vi "EDS test 01_with motor and Firebase with all sensors.vi"() -> ()   [LabVIEW 2020]
uses:
  <vilib>/DAQmx/read.llb/DAQmx Read (Digital Bool 1Line 1Point).vi
  <vilib>/DAQmx/write.llb/DAQmx Write (Digital Bool 1Line 1Point).vi
  <vilib>/DAQmx/read.llb/DAQmx Read (Analog Wfm 1Chan 1Samp).vi
  <vilib>/Analysis/baseanly.llb/Mean (DBL).vi
  <vilib>/Instr/_visa.llb/VISA Configure Serial Port (Instr).vi
  <vilib>/DAQmx/create/channels.llb/DAQmx Create Channel (DI-Digital Input).vi
  <vilib>/DAQmx/create/channels.llb/DAQmx Create Channel (DO-Digital Output).vi
  <vilib>/DAQmx/create/channels.llb/DAQmx Create Channel (AI-Voltage-Basic).vi
  <vilib>/DAQmx/miscellaneous.llb/DAQmx Fill In Error Info.vi
  <vilib>/httpClient/PUTBuffer.vi
  <vilib>/httpClient/LabVIEWHTTPClient.lvlib
  <vilib>/Analysis/NI_AALBase.lvlib
panel:
  out "Custom Sensor * 25":dbl(graph)
  out "Custom Sensor":dbl
  out "Train Speed":string
  out "Trolley Speed":string
  out "Trolley Distance":dbl
  out "Elephant Distance":dbl
  out "IR and Force Sensor":bool
  out "Custom Sensor":waveform(dbl)(graph)
  out "error out":errorcluster
  out "Concatenated String":string
  out "read buffer":string
  in  "stop":bool
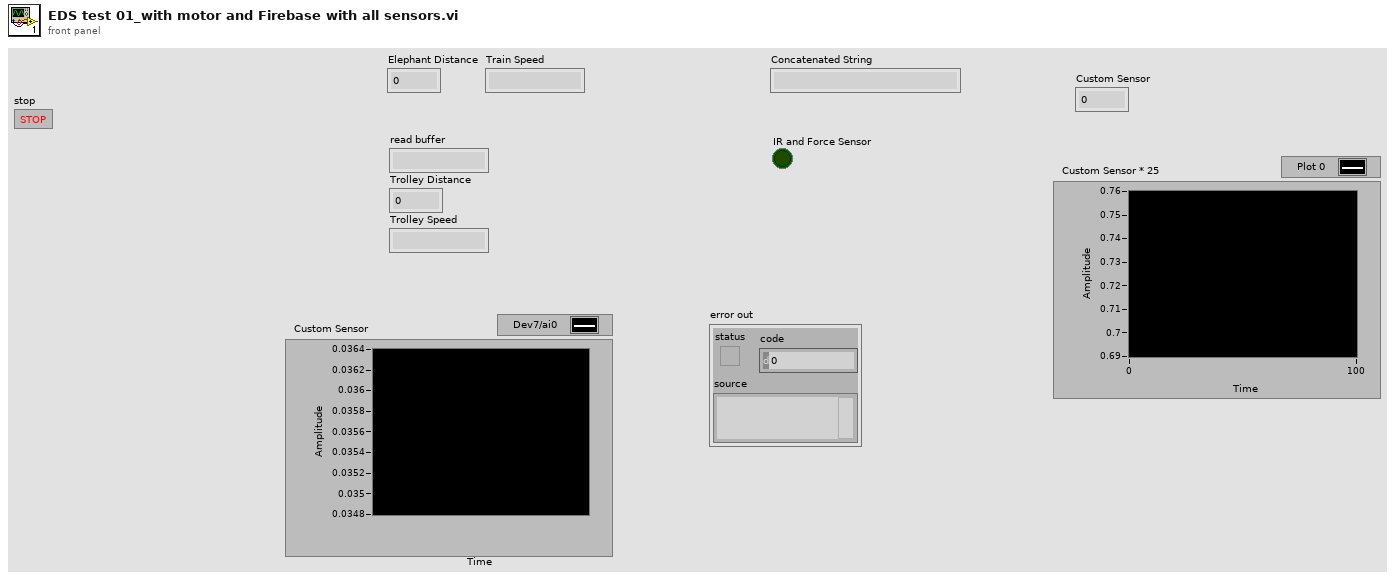
[diagram p1: front panel]
types:
  T1 = typedef "LabVIEWHTTPClient.lvlib/ClientHandle.ctl" = refnum<k1>
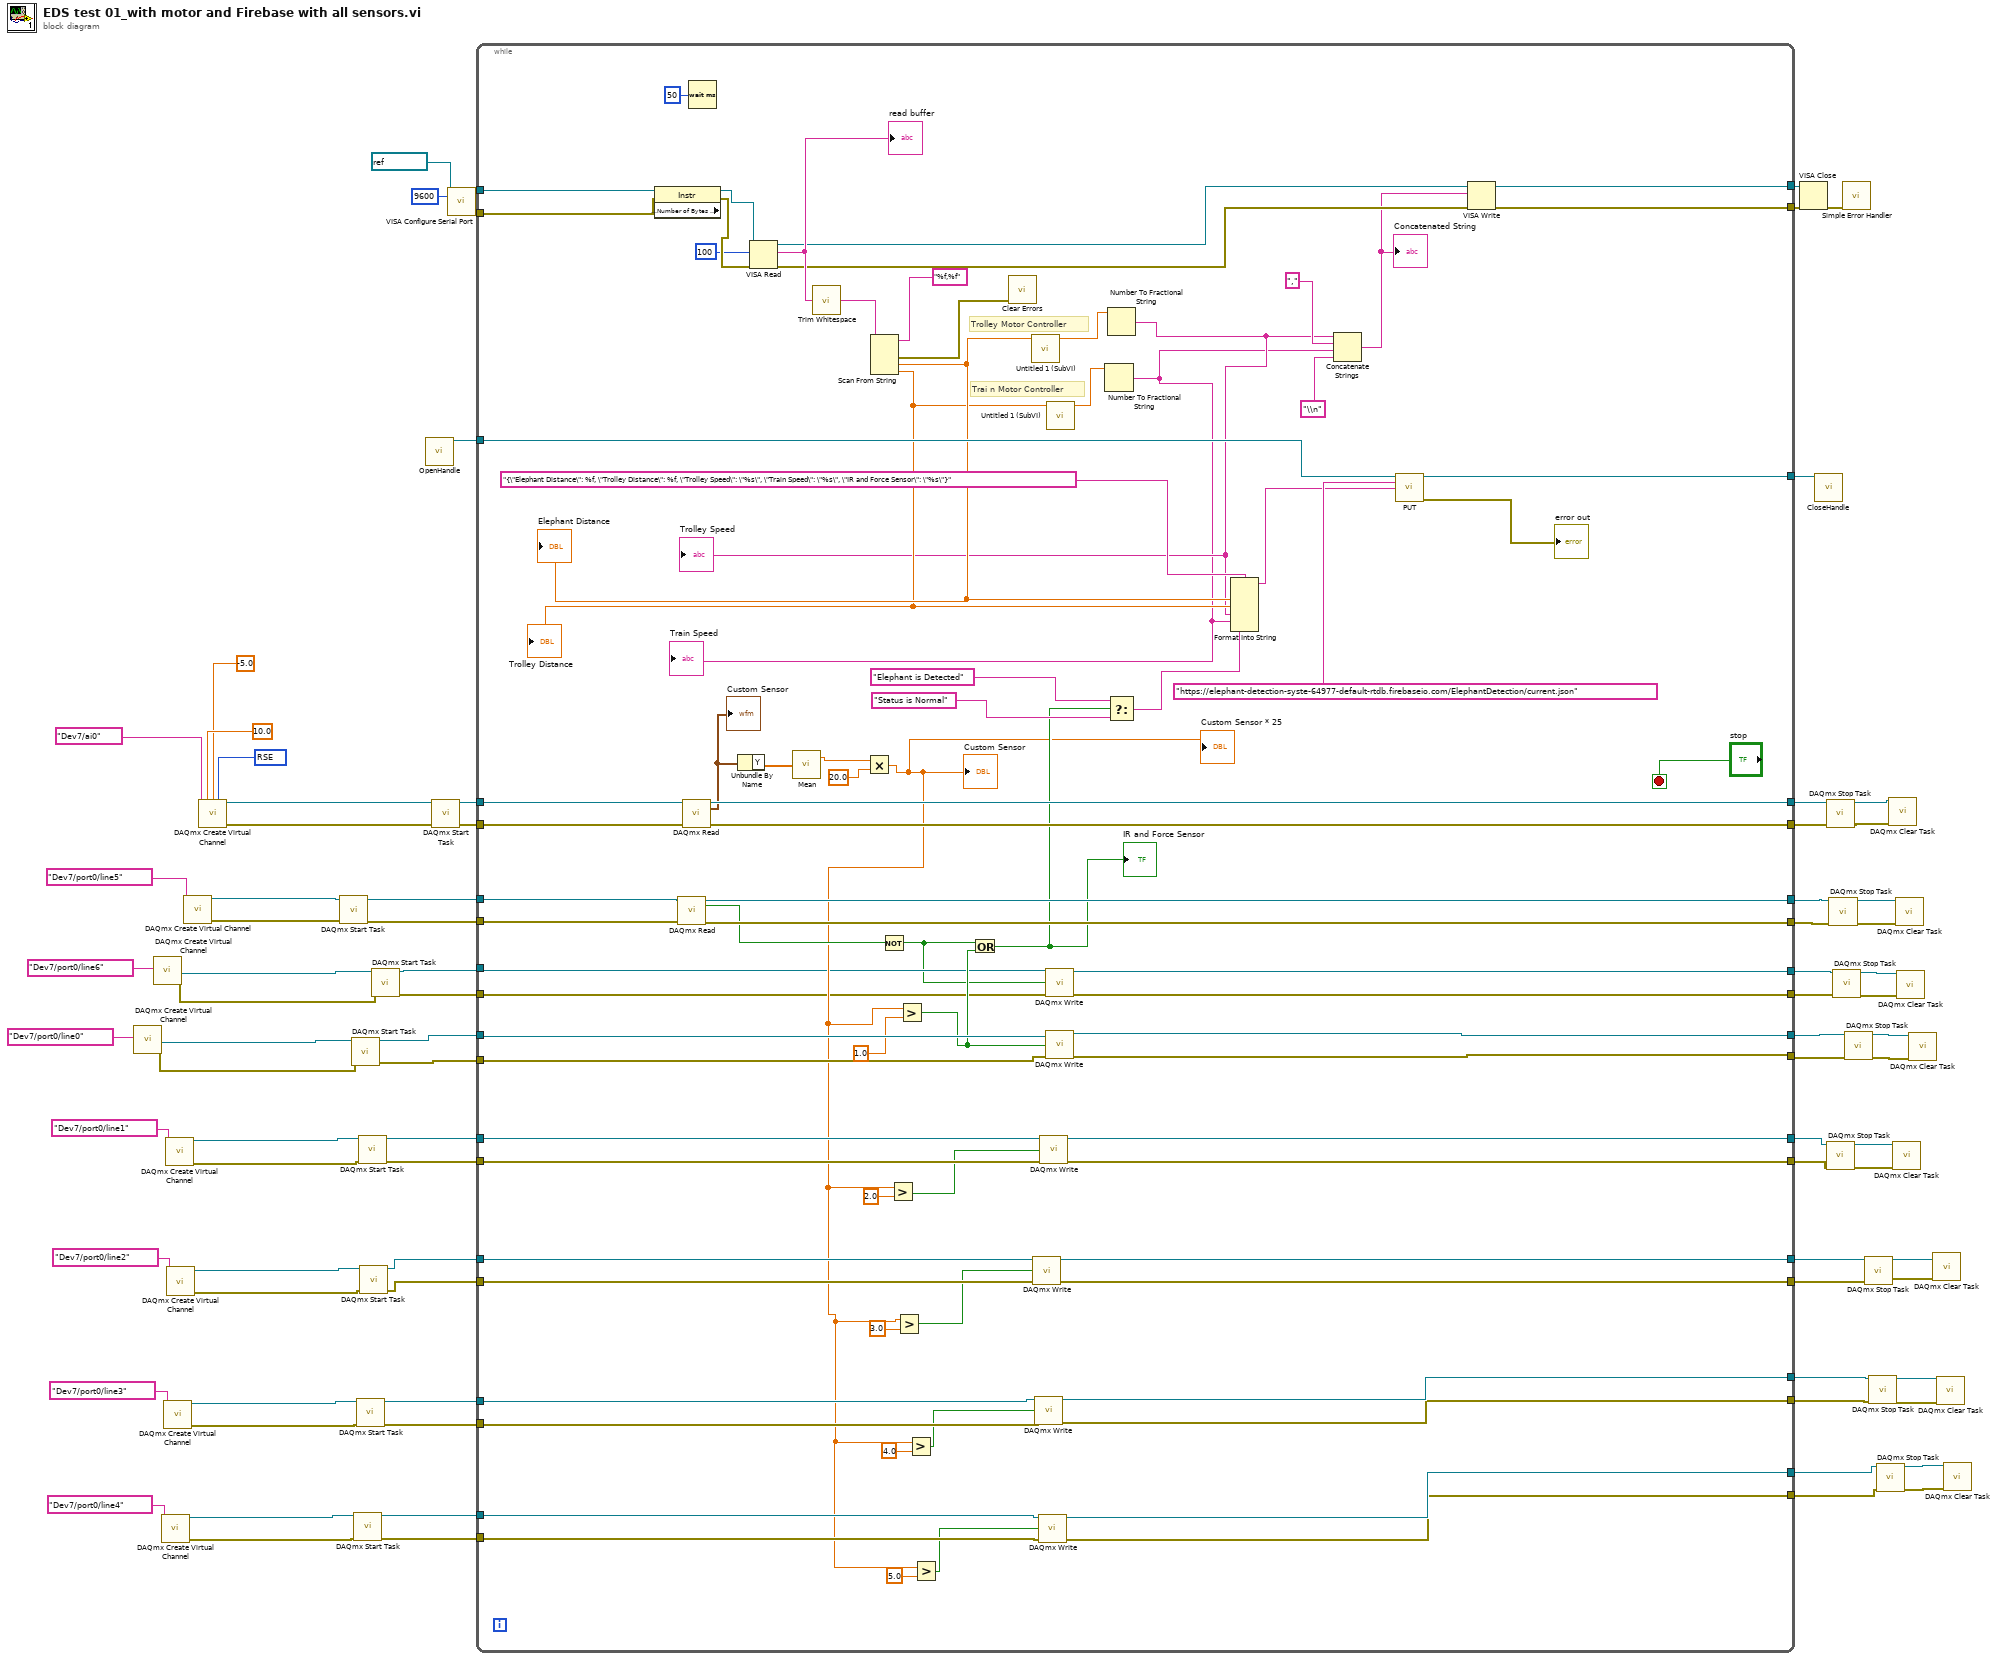
[diagram p0: block diagram]
diagram:
  w48 = 10083 items=["Default"=-1, "RSE"=10083, "NRSE"=10078, "Differential"=10106, "Pseudodifferential"=12529] ("input terminal configuration")
  n1 = call-poly <vilib>:"DAQmx Create Virtual Channel.vi"("lines"=tag "Dev7/port0/line0") -> ("task out"=w57:refnum<k21>, "error out"=w55:errorcluster)  [unwired: 13 in]
  n2 = call-poly <vilib>:"DAQmx Create Virtual Channel.vi"("lines"=tag "Dev7/port0/line6") -> ("task out"=w9:refnum<k21>, "error out"=w8:errorcluster)  [unwired: 13 in]
  n3 = call-poly <vilib>:"DAQmx Create Virtual Channel.vi"("lines"=tag "Dev7/port0/line4") -> ("task out"=w24:refnum<k21>, "error out"=w23:errorcluster)  [unwired: 13 in]
  n4 = call-poly <vilib>:"DAQmx Create Virtual Channel.vi"("lines"=tag "Dev7/port0/line3") -> ("task out"=w27:refnum<k21>, "error out"=w26:errorcluster)  [unwired: 13 in]
  n5 = call-poly <vilib>:"DAQmx Create Virtual Channel.vi"("lines"=tag "Dev7/port0/line1") -> ("task out"=w47:refnum<k21>, "error out"=w46:errorcluster)  [unwired: 13 in]
  n6 = call-poly <vilib>:"DAQmx Create Virtual Channel.vi"("lines"=tag "Dev7/port0/line2") -> ("task out"=w44:refnum<k21>, "error out"=w43:errorcluster)  [unwired: 13 in]
  n7 = call-poly <vilib>:"DAQmx Create Virtual Channel.vi"("lines"=tag "Dev7/port0/line5") -> ("task out"=w65:refnum<k21>, "error out"=w64:errorcluster)  [unwired: 13 in]
  n8 = call-poly <vilib>:"DAQmx Create Virtual Channel.vi"("maximum value"=10.0, "minimum value"=-5.0, "input terminal configuration"=w48, "physical channels"=tag "Dev7/ai0") -> ("task out"=w29:refnum<k21>, "error out"=w28:errorcluster)  [unwired: 10 in]
  n9 = call <vilib>:"DAQmx Start Task.vi"("task/channels in"=w65, "error in"=w64) -> ("task out"=w63:refnum<k21>, "error out"=w62:errorcluster)  [unwired: 12 in]
  n10 = call <vilib>:"DAQmx Start Task.vi"("task/channels in"=w57, "error in"=w55) -> ("task out"=w56:refnum<k21>, "error out"=w54:errorcluster)  [unwired: 12 in]
  n11 = call <vilib>:"DAQmx Start Task.vi"("task/channels in"=w24, "error in"=w23) -> ("task out"=w11:refnum<k21>, "error out"=w10:errorcluster)  [unwired: 12 in]
  n12 = call <vilib>:"DAQmx Start Task.vi"("task/channels in"=w27, "error in"=w26) -> ("task out"=w13:refnum<k21>, "error out"=w12:errorcluster)  [unwired: 12 in]
  n13 = call <vilib>:"DAQmx Start Task.vi"("task/channels in"=w47, "error in"=w46) -> ("task out"=w41:refnum<k21>, "error out"=w40:errorcluster)  [unwired: 12 in]
  n14 = call <vilib>:"DAQmx Start Task.vi"("task/channels in"=w44, "error in"=w43) -> ("task out"=w39:refnum<k21>, "error out"=w38:errorcluster)  [unwired: 12 in]
  n15 = call <vilib>:"DAQmx Start Task.vi"("task/channels in"=w9, "error in"=w8) -> ("task out"=w6:refnum<k21>, "error out"=w5:errorcluster)  [unwired: 12 in]
  n16 = call <vilib>:"OpenHandle.vi"() -> ("client handle out"=w77:T1)  [unwired: 14 in, 1 out]
  n17 = call <vilib>:"DAQmx Start Task.vi"("task/channels in"=w29, "error in"=w28) -> ("task out"=w75:refnum<k21>, "error out"=w70:errorcluster)  [unwired: 12 in]
  n18 = call-poly "VISA Configure Serial Port"("VISA resource name"=refnum<visa-resource-name> "COM3", "baud rate (9600)"=u32 9600) -> ("VISA resource name out"=w82:refnum<visa-resource-name>, "error out"=w81:errorcluster)  [unwired: 12 in]
  n19 = while {
    tunnel: w82 -> [w167]
    tunnel: w81 -> [w166]
    tunnel: [w152] -> w79
    tunnel: [w151] -> w78
    tunnel: w77 -> [w140]
    tunnel: [w139] -> w76
    tunnel: w75 -> [w134]
    tunnel: [w133] -> w74
    tunnel: [w132] -> w71
    tunnel: w70 -> [w131]
    tunnel: w63 -> [w130]
    tunnel: w62 -> [w129]
    tunnel: [w128] -> w61
    tunnel: [w127] -> w58
    tunnel: w56 -> [w126]
    tunnel: w54 -> [w125]
    tunnel: [w124] -> w53
    tunnel: [w123] -> w52
    tunnel: w41 -> [w117]
    tunnel: w40 -> [w116]
    tunnel: w39 -> [w115]
    tunnel: w38 -> [w114]
    tunnel: [w113] -> w33
    tunnel: [w112] -> w32
    tunnel: [w111] -> w31
    tunnel: [w110] -> w30
    tunnel: [w102] -> w17
    tunnel: [w101] -> w16
    tunnel: [w100] -> w15
    tunnel: [w99] -> w14
    tunnel: w13 -> [w97]
    tunnel: w12 -> [w96]
    tunnel: w11 -> [w95]
    tunnel: w10 -> [w94]
    tunnel: w6 -> [w89]
    tunnel: w5 -> [w88]
    tunnel: [w86] -> w2
    tunnel: [w85] -> w1
    stop <- "stop" stop-if-true
    # "Trai n Motor Controller"
    # "Trolley Motor Controller"
    n20 = property class="Instr" props=["Serial Settings:Number of Bytes at Serial Port"](reference=w167, error in=w166) -> (reference out=w162:refnum<visa-resource-name>, error out=w163:errorcluster)  [unwired: 1 out]
    n21 = call-poly <vilib>:"DAQmx Read.vi"("task/channels in"=w130, "error in"=w129) -> ("task out"=w128:refnum<k21>, "data"=w122:bool, "error out"=w127:errorcluster)  [unwired: 11 in]
    n22 = call-poly <vilib>:"DAQmx Read.vi"("task/channels in"=w134, "error in"=w131) -> ("task out"=w133:refnum<k21>, "data"=w121:waveform(dbl), "error out"=w132:errorcluster)  [unwired: 11 in]
    "Custom Sensor" <- w121
    n23 = Wait (ms)(milliseconds to wait=u32 50) -> ()  [unwired: 1 out]
    n24 = Unbundle By Name(w121) -> ("Y"=w120:dbl[])
    n25 = VISA Read(VISA resource name=w162, byte count=u32 100, error in (no error)=w163) -> (VISA resource name out=w154:refnum<visa-resource-name>, read buffer=w161:string, error out=w153:errorcluster)  [unwired: 1 out]
    "read buffer" <- w161
    n26 = call-poly <vilib>:"Mean.vi"("X"=w120) -> ("mean"=w119:dbl)  [unwired: 1 out]
    n27 = call <vilib>:"Trim Whitespace.vi"("string"=w161) -> ("trimmed string"=w160:string)  [unwired: 1 in]
    n28 = Multiply(x=w119, y=20.0) -> (x*y=w90:dbl)
    "Custom Sensor" <- w90
    "Custom Sensor * 25" <- w90
    n29 = Scan From String "Scan From String"(format string="%f,%f", input string=w160) -> (error out=w158:errorcluster, output 1=w138:dbl, output 2=w137:dbl)  [unwired: 4 in, 2 out]
    "Elephant Distance" <- w138
    "Trolley Distance" <- w137
    n30 = Not(x=w122) -> (.not. x?=w87:bool)
    n31 = Greater?(x=w90, y=2.0) -> (0:w105:bool)
    n32 = Greater?(x=w90, y=3.0) -> (0:w106:bool)
    n33 = Greater?(x=w90, y=1.0) -> (0:w104:bool)
    n34 = Greater?(x=w90, y=4.0) -> (0:w92:bool)
    n35 = Greater?(x=w90, y=5.0) -> (0:w91:bool)
    n36 = Or(x=w87, y=w104) -> (x .or. y?=w103:bool)
    "IR and Force Sensor" <- w103
    n37 = call <vilib>:"Clear Errors.vi"("error in (no error)"=w158) -> ()  [unwired: 5 in, 2 out]
    n38 = call "Untitled 1 (SubVI).vi"("Ultrasonic 01"=w138) -> ("Numeric"=w156:dbl)  [unwired: 10 in]
    n39 = call-poly <vilib>:"DAQmx Write.vi"("task/channels in"=w115, "data"=w106, "error in"=w114) -> ("task out"=w111:refnum<k21>, "error out"=w110:errorcluster)  [unwired: 10 in, 1 out]
    n40 = call-poly <vilib>:"DAQmx Write.vi"("task/channels in"=w97, "data"=w92, "error in"=w96) -> ("task out"=w102:refnum<k21>, "error out"=w101:errorcluster)  [unwired: 10 in, 1 out]
    n41 = call-poly <vilib>:"DAQmx Write.vi"("task/channels in"=w95, "data"=w91, "error in"=w94) -> ("task out"=w100:refnum<k21>, "error out"=w99:errorcluster)  [unwired: 10 in, 1 out]
    n42 = call-poly <vilib>:"DAQmx Write.vi"("task/channels in"=w117, "data"=w105, "error in"=w116) -> ("task out"=w113:refnum<k21>, "error out"=w112:errorcluster)  [unwired: 10 in, 1 out]
    n43 = call-poly <vilib>:"DAQmx Write.vi"("task/channels in"=w89, "data"=w87, "error in"=w88) -> ("task out"=w86:refnum<k21>, "error out"=w85:errorcluster)  [unwired: 10 in, 1 out]
    n44 = call-poly <vilib>:"DAQmx Write.vi"("task/channels in"=w126, "data"=w104, "error in"=w125) -> ("task out"=w124:refnum<k21>, "error out"=w123:errorcluster)  [unwired: 10 in, 1 out]
    n45 = call "Untitled 1 (SubVI).vi"("Ultrasonic 01"=w137) -> ("Numeric"=w155:dbl)  [unwired: 10 in]
    n46 = Number To Fractional String(number=w155) -> (F-format string=w135:string)  [unwired: 3 in]
    "Train Speed" <- w135
    n47 = Number To Fractional String(number=w156) -> (F-format string=w136:string)  [unwired: 3 in]
    "Trolley Speed" <- w136
    n48 = Select(t="Elephant is Detected" ("format string"), s=w103, f="Status is Normal" ("format string")) -> (s? t:f=w145:string)
    n49 = Format Into String(format string="{\"Elephant Distance\": %f, \"Trolley Distance\": %f, \"Trolley Speed\": \"%s\", \"Train Speed\": \"%s\", \"IR and Force Sensor\": \"%s\"}", w138, w137, w136, w135, w145) -> (resulting string=w142:string)  [unwired: 2 in, 1 out]
    n50 = Concatenate Strings "Concatenate Strings"(w136, ",", w135, "\\n") -> (w150:string)
    "Concatenated String" <- w150
    n51 = call-poly <vilib>:"PUT.vi"("client handle"=w140, "url"="https://elephant-detection-syste-64977-default-rtdb.firebaseio.com/ElephantDetection/current.json", "buffer"=w142) -> ("client handle out"=w139:T1, "error out"=→"error out":errorcluster)  [unwired: 9 in, 2 out]
    n52 = VISA Write(VISA resource name=w154, write buffer=w150, error in (no error)=w153) -> (VISA resource name out=w152:refnum<visa-resource-name>, error out=w151:errorcluster)  [unwired: 1 out]
  }
  n53 = VISA Close(VISA resource name=w79, error in (no error)=w78) -> (error out=w80:errorcluster)
  n54 = call <vilib>:"CloseHandle.vi"("client handle"=w76) -> ()  [unwired: 14 in, 1 out]
  n55 = call <vilib>:"DAQmx Stop Task.vi"("task/channels in"=w74, "error in"=w71) -> ("task out"=w73:refnum<k21>, "error out"=w72:errorcluster)  [unwired: 12 in]
  n56 = call <vilib>:"DAQmx Stop Task.vi"("task/channels in"=w33, "error in"=w32) -> ("task out"=w37:refnum<k21>, "error out"=w36:errorcluster)  [unwired: 12 in]
  n57 = call <vilib>:"DAQmx Stop Task.vi"("task/channels in"=w61, "error in"=w58) -> ("task out"=w60:refnum<k21>, "error out"=w59:errorcluster)  [unwired: 12 in]
  n58 = call <vilib>:"DAQmx Stop Task.vi"("task/channels in"=w2, "error in"=w1) -> ("task out"=w4:refnum<k21>, "error out"=w3:errorcluster)  [unwired: 12 in]
  n59 = call <vilib>:"Simple Error Handler.vi"("error in (no error)"=w80) -> ()  [unwired: 4 in, 5 out]
  n60 = call <vilib>:"DAQmx Stop Task.vi"("task/channels in"=w53, "error in"=w52) -> ("task out"=w51:refnum<k21>, "error out"=w50:errorcluster)  [unwired: 12 in]
  n61 = call <vilib>:"DAQmx Stop Task.vi"("task/channels in"=w31, "error in"=w30) -> ("task out"=w35:refnum<k21>, "error out"=w34:errorcluster)  [unwired: 12 in]
  n62 = call <vilib>:"DAQmx Stop Task.vi"("task/channels in"=w17, "error in"=w16) -> ("task out"=w21:refnum<k21>, "error out"=w20:errorcluster)  [unwired: 12 in]
  n63 = call <vilib>:"DAQmx Stop Task.vi"("task/channels in"=w15, "error in"=w14) -> ("task out"=w19:refnum<k21>, "error out"=w18:errorcluster)  [unwired: 12 in]
  n64 = call <vilib>:"DAQmx Clear Task.vi"("task in"=w73, "error in"=w72) -> ()  [unwired: 13 in, 1 out]
  n65 = call <vilib>:"DAQmx Clear Task.vi"("task in"=w37, "error in"=w36) -> ()  [unwired: 13 in, 1 out]
  n66 = call <vilib>:"DAQmx Clear Task.vi"("task in"=w60, "error in"=w59) -> ()  [unwired: 13 in, 1 out]
  n67 = call <vilib>:"DAQmx Clear Task.vi"("task in"=w4, "error in"=w3) -> ()  [unwired: 13 in, 1 out]
  n68 = call <vilib>:"DAQmx Clear Task.vi"("task in"=w51, "error in"=w50) -> ()  [unwired: 13 in, 1 out]
  n69 = call <vilib>:"DAQmx Clear Task.vi"("task in"=w35, "error in"=w34) -> ()  [unwired: 13 in, 1 out]
  n70 = call <vilib>:"DAQmx Clear Task.vi"("task in"=w21, "error in"=w20) -> ()  [unwired: 13 in, 1 out]
  n71 = call <vilib>:"DAQmx Clear Task.vi"("task in"=w19, "error in"=w18) -> ()  [unwired: 13 in, 1 out]
